vi "Trigger Channel.vi"(8 "error in":errorcluster, 11 "Node Ptr":T1 format="%.0x") -> (0 "error out":errorcluster)   [LabVIEW 2020, in "AIM MIL-STD-1553 System Explorer.lvlib" / "Implementation.lvlib"]
uses:
  Implementation.lvlib
  <vilib>/NI VeriStand/Custom Device API/Custom Device API.lvlib
  <vilib>/NI VeriStand/Custom Device API/Custom Device Channel Type.ctl
  Scripting/AIM MIL-STD-1553 Scripting.lvlib
  <vilib>/NI VeriStand/Custom Device API/Custom Device Item Ref.ctl
panel:
  out "acyclic buffer ID":string caption="Acyclic Buffer ID"
  out "Channel Settings":string[][](table)
  in  "Default Value":dbl
  in  "SHDocVw.IWebBrowser":refnum<k7>(container)
  in  "General Header":cluster{"Section Name":string}={"Section Name"="MIL-STD-1553 - Trigger Channel"}
  in  "Description":string
  out "Name":string
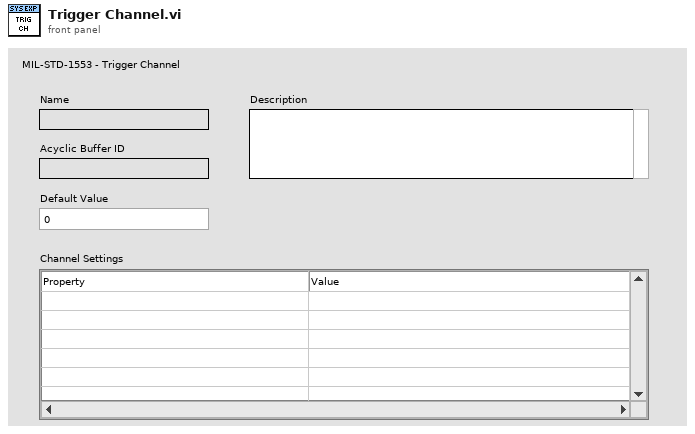
[diagram p1: front panel]
types:
  T1 = typedef "Custom Device API.lvlib/Custom Device Item Ref.ctl" = u64
  T2 = typedef "Custom Device API.lvlib/Custom Device Channel Type.ctl" = enum16{"Input", "Output"}
  T3 = typedef "Custom Device API.lvlib/Custom Device Channel.ctl" = cluster{"Type":T2, "Units":string, "Default Value":dbl, "Faultable":bool, "Scalable":bool}
  T4 = typedef "Custom Device API.lvlib/Custom Device Commands.ctl" = enum16{"Default", "Item renamed", "Shutdown", "Dynamic button pressed"}
  T5 = typedef "Custom Device API.lvlib/Custom Device Item Info.ctl" = cluster{"Name":string, "Is Channel":bool, "GUID":string, "Is Waveform":bool}
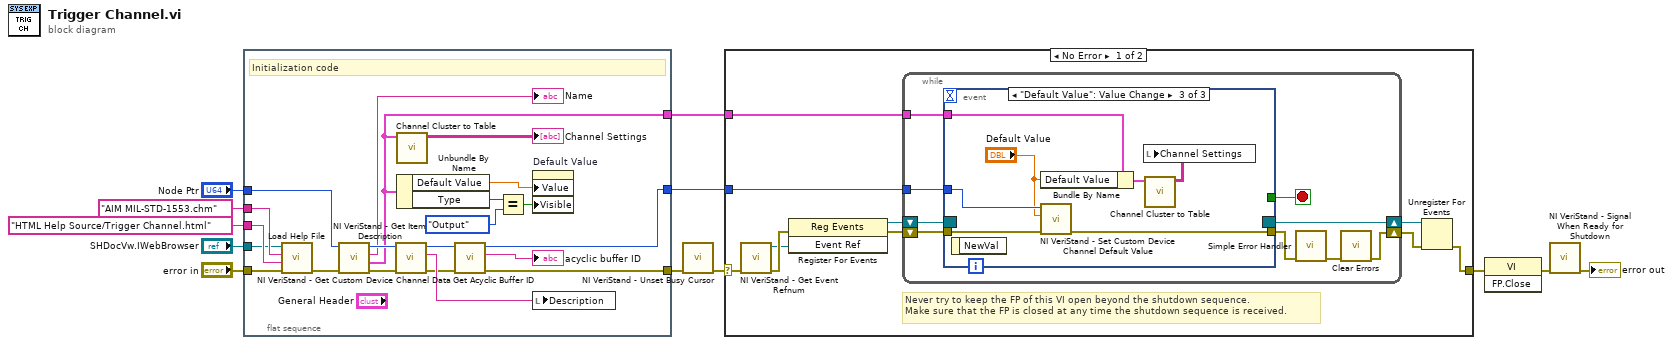
[diagram p0: block diagram]
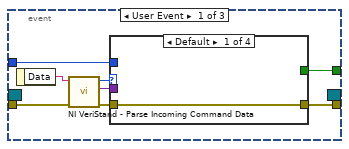
[diagram p2: hidden frame]
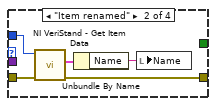
[diagram p3: hidden frame]
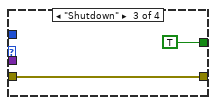
[diagram p4: hidden frame]
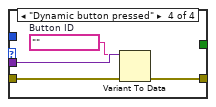
[diagram p5: hidden frame]
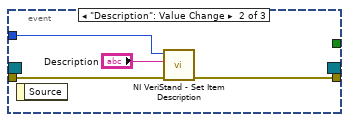
[diagram p6: hidden frame]
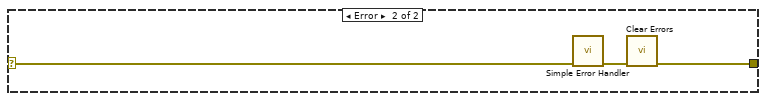
[diagram p7: hidden frame]
diagram:
  n1 = flat-sequence "Initialization code" {
    tunnel: "error in" -> [w32]
    tunnel: "Node Ptr" -> [w28]
    tunnel: [w13] -> w8
    tunnel: [w15] -> w5
    tunnel: "SHDocVw.IWebBrowser" -> [w29]
    tunnel: "HTML Help Source/Trigger Channel.html" ("CD_CHM_Section") -> [w31]
    tunnel: "AIM MIL-STD-1553.chm" ("CD_CHM_FileName") -> [w30]
    tunnel: [w18] -> w1
    frame #0 {
      # "Initialization code"
      n2 = call "Load Help File.vi"("error in (no error)"=w32, "HTML File to Load"=w31, "Main CHM File"=w30, "Browser"=w29) -> ("error out"=w26:errorcluster)  [unwired: 7 in]
      n3 = call <vilib>:"NI VeriStand - Get Custom Device Channel Data.vi"("error in (no error)"=w26, "Channel Ref in"=w28) -> ("error out"=w27:errorcluster, "Channel"=w18:T3, "Channel Name"=→"Name":string, "Channel Ref out"=w22:T1)  [unwired: 4 in, 2 out]
      n4 = call <vilib>:"NI VeriStand - Get Item Description.vi"("error in (no error)"=w27, "Item Ref in"=w22) -> ("error out"=w14:errorcluster, "Description"=w33:string, "Item Ref out"=w16:T1)  [unwired: 7 out]
      n5 = call "Channel Cluster to Table.vi"("channel settings"=w18) -> ("channel settings table"=→"Channel Settings":string[][])  [unwired: 10 in]
      n6 = Unbundle By Name(w18) -> ("Default Value"=w19:dbl, "Type"=w25:T2)
      n7 = call "Get Acyclic Buffer ID.vi"("error in"=w14, "acyclic frame trigger"=w16) -> ("error out"=w13:errorcluster, "acyclic buffer id"=→"acyclic buffer ID":string, "acyclic frame trigger out"=w15:T1)  [unwired: 7 in]
      n8 = Equal?(x=w25, y=Custom_Device_Channel_Type."Output" ("x")) -> (x = y?=w23:bool)
      n9 = property on="Default Value" class="DigNum (strict)"("Value"=w19, "Visible"=w23) -> ()  [unwired: 2 in, 2 out]
      n10 = local write "Description"(w33) -> ()
    }
  }
  n11 = call <vilib>:"NI VeriStand - Unset Busy Cursor.vi"("error in (no error)"=w8) -> ("error out"=w7:errorcluster)  [unwired: 10 out]
  n12 = case shown="No Error" w7 {
    selector: w7 -> [w35 w86]
    tunnel: [w40 w84] -> w12
    tunnel: w5 -> [w36 _]
    tunnel: w1 -> [w34 _]
    frame No Error {
      # "Never try to keep the FP of this VI open beyond the shutdown sequence.\nMake sure that the FP is closed at any time the shutdown sequence is received."
      n13 = call <vilib>:"NI VeriStand - Get Event Refnum.vi"("error in (no error)"=w35) -> ("error out"=w43:errorcluster, "Event Ref"=w39:refnum<user-event>)  [unwired: 9 out]
      n14 = register-events(error in=w43, w39) -> (reference out=w37:refnum<event-registration>, error out=w38:errorcluster)  [unwired: 1 in]
      n15 = while {
        tunnel: w36 -> [w48]
        shift-right: [w45] -> w41
        shift-left: w38 -> [w51]
        shift-right: [w52] -> w42
        shift-left: w37 -> [w50]
        tunnel: w34 -> [w44]
        stop <- w49 stop-if-true
        n16 = event shown="[2] \"Default Value\": Value Change" {
          selector: w50 -> [_ _ _]
          dyn-events: [_ _ _] -> w52
          timeout: _ -> [_ _ _]
          tunnel: w51 -> [w60 w75 w83]
          tunnel: [w57 _ _] -> w49
          tunnel: [w56 w74 w82] -> w47
          tunnel: w48 -> [w55 w76 w81]
          tunnel: w44 -> [_ _ w79]
          event User Event {
            n17 = event-data() -> ("Data"=w53:string)  [unwired: 1 out]
            n18 = call <vilib>:"NI VeriStand - Parse Incoming Command Data.vi"("error in (no error)"=w60, "Incoming data"=w53) -> ("error out"=w59:errorcluster, "Outgoing data"=w54:variant, "Action"=w58:T4)  [unwired: 7 out]
            n19 = case shown="Default" w58 {
              tunnel: w59 -> [w61 w66 w67 w72]
              tunnel: [_ _ TRUE _] -> w57
              tunnel: [w61 w63 w67 w69] -> w56
              tunnel: w55 -> [_ w65 _ _]
              tunnel: w54 -> [_ _ _ w71]
              frame Default {
              }
              frame "Item renamed" {
                n20 = call <vilib>:"NI VeriStand - Get Item Data.vi"("error in (no error)"=w66, "Item Ref in"=w65) -> ("error out"=w63:errorcluster, "Item Info"=w64:T5)  [unwired: 8 out]
                n21 = Unbundle By Name(w64) -> ("Name"=w62:string)
                n22 = local write "Name"(w62) -> ()
              }
              frame "Shutdown" {
              }
              frame "Dynamic button pressed" {
                w70 = ""  # Button ID
                n23 = Variant To Data(error in=w72, type=w70, Variant=w71) -> (error out=w69:errorcluster)  [unwired: 1 out]
              }
            }
          }
          event "Description": Value Change {
            n24 = event-data() -> ()  [unwired: 2 out]
            n25 = call <vilib>:"NI VeriStand - Set Item Description.vi"("error in (no error)"=w75, "Description"="Description", "Item Ref in"=w76) -> ("error out"=w74:errorcluster)  [unwired: 8 out]
          }
          event "Default Value": Value Change {
            n26 = event-data() -> ()  [unwired: 2 out]
            n27 = Bundle By Name(cluster=w79, "Default Value"="Default Value") -> (w77:T3)
            n28 = call <vilib>:"NI VeriStand - Set Custom Device Channel Default Value.vi"("error in (no error)"=w83, "Default Value"="Default Value", "Channel Ref in"=w81) -> ("error out"=w82:errorcluster)  [unwired: 7 in, 1 out]
            n29 = call "Channel Cluster to Table.vi"("channel settings"=w77) -> ("channel settings table"=w80:string[][])  [unwired: 10 in]
            n30 = local write "Channel Settings"(w80) -> ()
          }
        }
        n31 = call <vilib>:"Simple Error Handler.vi"("error in (no error)"=w47) -> ("error out"=w46:errorcluster)  [unwired: 1 in, 7 out]
        n32 = call <vilib>:"Clear Errors.vi"("error in (no error)"=w46) -> ("error out"=w45:errorcluster)  [unwired: 1 in, 5 out]
      }
      n33 = Unregister For Events(event registration refnum=w42, error in=w41) -> (error out=w40:errorcluster)
    }
    frame Error {
      n34 = call <vilib>:"Simple Error Handler.vi"("error in (no error)"=w86) -> ("error out"=w85:errorcluster)  [unwired: 1 in, 7 out]
      n35 = call <vilib>:"Clear Errors.vi"("error in (no error)"=w85) -> ("error out"=w84:errorcluster)  [unwired: 1 in, 5 out]
    }
  }
  n36 = invoke class="VI" method="FP.Close"(error in=w12) -> (error out=w11:errorcluster)  [unwired: 2 in, 2 out]
  n37 = call <vilib>:"NI VeriStand - Signal When Ready for Shutdown.vi"("error in (no error)"=w11) -> ("error out"=→"error out":errorcluster)  [unwired: 10 out]
